vi "app_kind_lua.vi"(5 "LuaVIEW reference":T1) -> (15 "error out":errorcluster)   [LabVIEW 2012]
doc: "Returns the \"kind\" application property enum. Under LabVIEW 7, it has as possible values: \"invalid app kind\", \"Development System\", \"Run Time System\", \"Student Edition\", \"Embedded LabVIEW\", \"Evaluation\", and \"Custom\". Note that future LabVIEW versions might add more kinds.\n\nThis function allows a script to perform actions that depend on how the application is deployed. For example, compare the result string to \"Development System\" and take actions particular to the development setup if equal, or actions particular to the built setup if not equal.\nResults:\nstr:kind"
uses:
  typedefs/t_LuaVIEW Reference.ctl
  subvis/private/LuaVIEW Push (string).vi
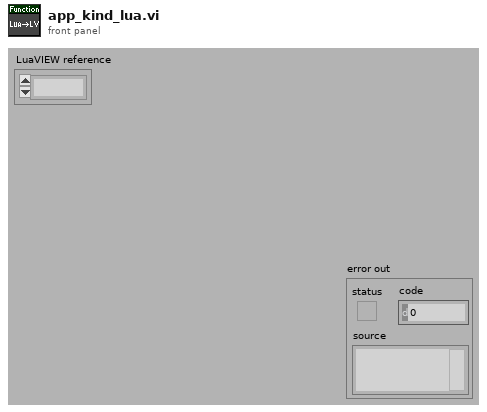
[diagram p1: front panel]
types:
  T1 = typedef "t_LuaVIEW Reference.ctl" = refnum<k1>
  T2 = enum32{"invalid app kind", "Development System", "Run Time System", "Student Edition", "Embedded LabVIEW", "Evaluation", "Custom"}
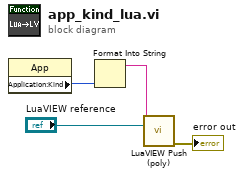
[diagram p0: block diagram]
diagram:
  n1 = property class="App"() -> ("Application:Kind"=w3:T2)  [unwired: 2 in, 2 out]
  n2 = Format Into String(w3) -> (resulting string=w4:string)  [unwired: 3 in, 1 out]
  n3 = call-poly "LuaVIEW Push (poly).vi"("string"=w4, "LuaVIEW reference in"="LuaVIEW reference") -> ("error out"=→"error out":errorcluster)  [unwired: 12 in, 1 out]
